vi "形态学操作.vi"() -> ()   [LabVIEW 2018]
doc: "This example shows how to use the Edge Tool in NI Vision. The Edge Tool finds edges (or sharp transitions in the pixels values) along a given line or ROI profile. The Edge Tool is a precursor function to many of the gauging and inspection tasks. For example, the location of the edges found along a line profile across an object can interpreted as the boundaries of the object whose dimensions have to be measured for a gauging application or the presence of a crack in the surface of an object for an inspection application."
uses:
  <vilib>/vision/NI_Vision_Development_Module.lvlib
panel:
  out "Src":T1(plugin-control)
  in  "Structuring Element":i32[][](array[numeric])=[[0, 1, 0], [1, 1, 1], [0, 0, 0]]
  in  "Hexa Pixel?":bool
  in  "# of iterations":i32=1
  in  "Operation":u16(ring) items=["AutoM", "Close", "Dilate", "Erode", "Gradient", "Gradient out", "Gradient in", "Hit miss", "Open", "PClose", "POpen", "Thick", "Thin"]
  out "Dst":T1(plugin-control)
  in  "Stop":bool
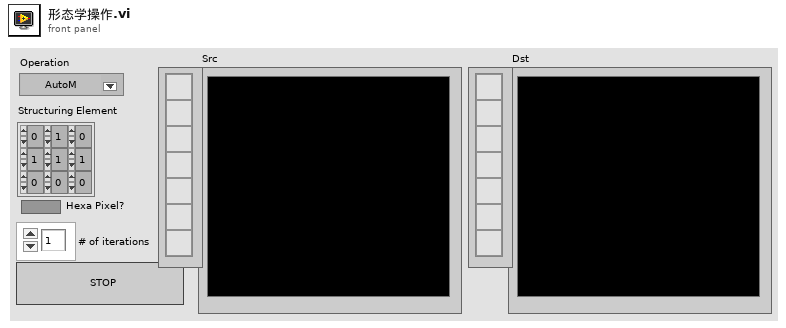
[diagram p1: front panel]
types:
  T1 = typedef "IMAQ Image.ctl" = refnum<image>
  T2 = typedef "Image Type" = u32
  T3 = cluster{"Hexa Pixel?":bool, "Operation":u16, "Structuring Element":i32[][], "# of iterations":i32}
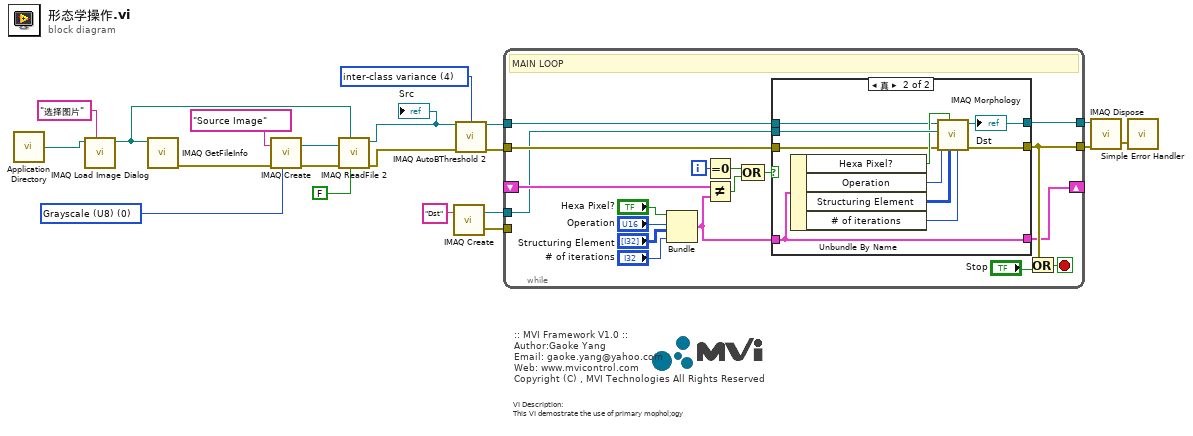
[diagram p0: block diagram]
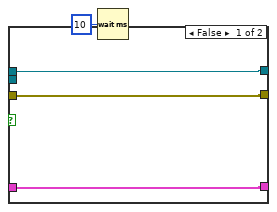
[diagram p2: hidden frame]
diagram:
  w4 = T2 0 items=["Grayscale (U8)", "Grayscale (I16)", "Grayscale (SGL)", "Complex (CSG)", "RGB (U32)", "HSL (U32)", "RGB (U64)", "Grayscale (U16)"] ("Image Type")
  w14 = 4 items=["clustering", "entropy", "metric", "moments", "inter-class variance"] ("Method")
  # "VI Description:\nThis VI demostrate the use of primary mophol;ogy"
  # ":: MVI Framework V1.0 ::\nAuthor:Gaoke Yang\nEmail: gaoke.yang@yahoo.com\nWeb: www.mvicontrol.com\nCopyright (C) , MVI Technologies All Rights Reserved"
  n1 = call <vilib>:"Application Directory.vi"() -> ("Application Directory"=w5:path)
  n2 = call "IMAQ Load Image Dialog"("Prompt"="选择图片" ("prompt"), "Start Path"=w5) -> ("Path"=w11:path)  [unwired: 7 in, 2 out]
  n3 = call "IMAQ GetFileInfo"("File Path"=w11) -> ("error out"=w9:errorcluster)  [unwired: 4 in, 6 out]
  n4 = call "IMAQ Create"("Image Name"="Source Image", "Image Type"=w4, "error in (no error)"=w9) -> ("New Image"=w7:T1, "error out"=w6:errorcluster)  [unwired: 2 in]
  n5 = call "IMAQ ReadFile 2"("Use File Path Image Type"=FALSE, "File Path"=w11, "error in (no error)"=w6, "Image"=w7) -> ("error out"=w1:errorcluster, "Image Out"=w2:T1)  [unwired: 3 in, 3 out]
  "Src" <- w2
  n6 = call "IMAQ Create"("Image Name"="Dst") -> ("New Image"=w16:T1, "error out"=w15:errorcluster)  [unwired: 4 in]
  n7 = call "IMAQ AutoBThreshold 2"("Image Src"=w2, "Method (clustering)"=w14, "error in (no error)"=w1) -> ("Image Dst Out"=w12:T1, "error out"=w13:errorcluster)  [unwired: 5 in, 6 out]
  n8 = while "MAIN LOOP" {
    tunnel: w12 -> [w37]
    tunnel: w13 -> [w38]
    tunnel: [w33] -> w20
    tunnel: [w34] -> w19
    shift-right: [w30] -> _
    shift-left: _ -> [w27]
    tunnel: w16 -> [w25]
    tunnel: w15 -> [_]
    i -> [w32]
    stop <- w35 stop-if-true
    # "MAIN LOOP"
    n9 = Bundle("Hexa Pixel?"="Hexa Pixel?", "Operation"="Operation", "Structuring Element"="Structuring Element", "# of iterations"="# of iterations") -> (w28:T3)  [unwired: 1 in]
    n10 = Equal To 0?(x=w32) -> (x = 0?=w29:bool)
    n11 = Not Equal?(x=w27, y=w28) -> (x != y?=w26:bool)
    n12 = Compound Arithmetic op=OR(w29, w26) -> (w31:bool)
    n13 = case shown="真" w31 {
      tunnel: w38 -> [w41 w43]
      tunnel: w37 -> [w42 w44]
      tunnel: [w42 w45] -> w34
      tunnel: [w41 w46] -> w33
      tunnel: [w39 w51] -> w30
      tunnel: w28 -> [w39 w51]
      tunnel: w25 -> [_ w52]
      frame False {
        n14 = Wait (ms)(milliseconds to wait=u32 10) -> ()  [unwired: 1 out]
      }
      frame True {
        n15 = Unbundle By Name(w51) -> ("Hexa Pixel?"=w47:bool, "Operation"=w48:u16, "Structuring Element"=w49:i32[][], "# of iterations"=w50:i32)
        n16 = call "IMAQ Morphology"("Number of iterations (1)"=w50, "Structuring Element"=w49, "Square/Hexa (Square)"=w47, "error in (no error)"=w43, "Operation"=w48, "Image Dst"=w52, "Image Src"=w44) -> ("error out"=w46:errorcluster, "Image Dst Out"=w45:T1)  [unwired: 3 in]
        "Dst" <- w45
      }
    }
    n17 = Or(x=w33, y="Stop") -> (x .or. y?=w35:bool)
  }
  n18 = call "IMAQ Dispose"("Image"=w19, "error in (no error)"=w20) -> ("error out"=w18:errorcluster)  [unwired: 4 in]
  n19 = call <vilib>:"Simple Error Handler.vi"("error in (no error)"=w18) -> ()  [unwired: 4 in, 5 out]
